vi "GUI Set Error To String.vi"(2 "error in (no error)":errorcluster, 3 "label(s) (status)":string="status") -> ()   [LabVIEW 2020]
doc: "Displays error in the string referenced by its label. The string object must be first registered by the SGUI lib."
uses:
  varilib/SGUI Assign Multiple Strings With Tags By Label.vi
  varilib/varilib.lvlib
panel:
  out "s? t:f":string
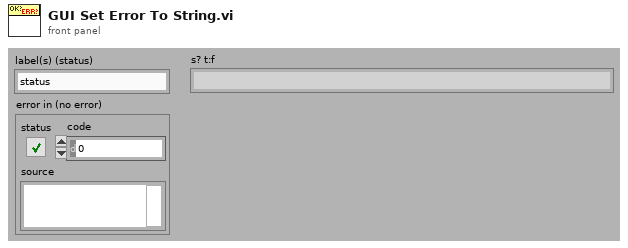
[diagram p1: front panel]
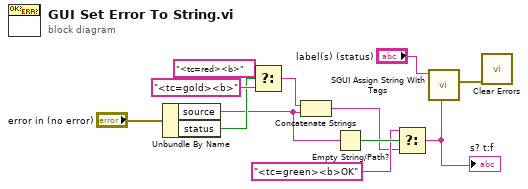
[diagram p0: block diagram]
diagram:
  n1 = Unbundle By Name("error in (no error)") -> ("source"=w3:string, "status"=w6:bool)
  n2 = Select(t="<tc=red><b>" ("string"), s=w6, f="<tc=gold><b>" ("string")) -> (s? t:f=w5:string)
  n3 = Concatenate Strings(w5, w3) -> (w1:string)
  n4 = Empty String/Path?(string/path=w3) -> (empty?=w4:bool)
  n5 = Select(t="<tc=green><b>OK" ("f"), s=w4, f=w1) -> (s? t:f=w11:string)
  "s? t:f" <- w11
  n6 = call-poly "SGUI Assign String With Tags.vi"("label(s) (empty)"="label(s) (status)", "string (empty)"=w11) -> ("error out"=w10:errorcluster)  [unwired: 8 in, 1 out]
  n7 = call <vilib>:"Clear Errors.vi"("error in (no error)"=w10) -> ()  [unwired: 5 in, 2 out]
